vi "ConfChannelMetodo.vi"(7 "Enable Channel (True)":bool=TRUE, 8 "error in (no error)":errorcluster, 10 "ConfigChannel":T1={"Probe Attenuation (10: 10X)"=10, "Vertical Range (10.0 V/div)"=10.0, "Vertical Offset (0.0 divs)"=0.0, "Bandwidth (0: MAX Bandwidth)"=0, "Channel (0: Channel 1)"=0, "Vertical Coupling (1: DC)"=1} {"Vertical Coupling (1: DC)" items=["AC", "DC", "Ground"]; "Channel (0: Channel 1)" items=["Channel 1", "Channel 2", "Channel 3", "Channel 4", "Math", "Reference A", "Reference B", "Reference C", "Reference D"]; "Bandwidth (0: MAX Bandwidth)" items=["MAX Bandwidth", "Unlimited"]; "Probe Attenuation (10: 10X)" items=["1"=1, "10"=10, "20"=20, "50"=50, "100"=100, "500"=500, "1000"=1000]}, 11 "Keysight in":refnum<class "Keysight.lvclass">) -> (0 "error out":errorcluster, 3 "Keysight out":refnum<class "Keysight.lvclass">)   [LabVIEW 2020, in "Keysight.lvclass"]
uses:
  Keysight.lvclass
  Keysight.lvclass/Keysight.ctl
  <instrlib>/Agilent 2000 3000 X-Series/Agilent 2000 3000 X-Series.lvlib
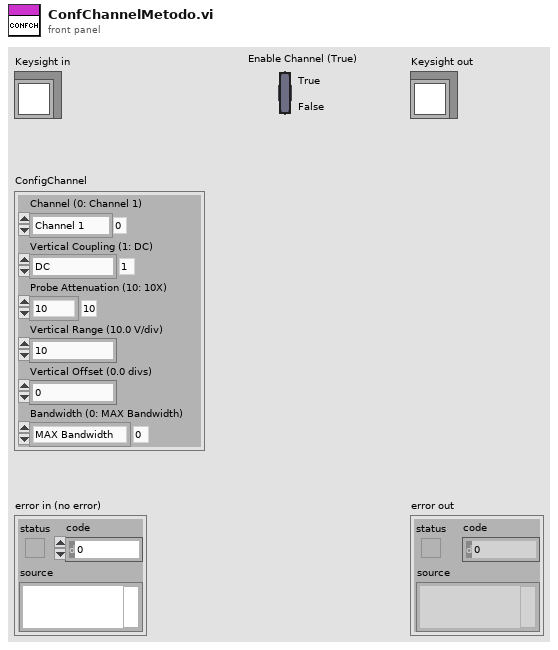
[diagram p1: front panel]
types:
  T1 = cluster{"Probe Attenuation (10: 10X)":i32, "Vertical Range (10.0 V/div)":dbl, "Vertical Offset (0.0 divs)":dbl, "Bandwidth (0: MAX Bandwidth)":i32, "Channel (0: Channel 1)":i32, "Vertical Coupling (1: DC)":i32}
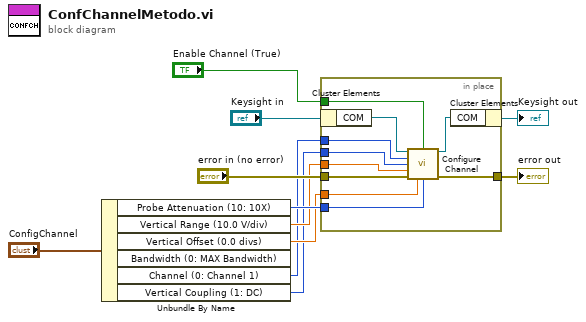
[diagram p0: block diagram]
diagram:
  n1 = Unbundle By Name("ConfigChannel") -> ("Probe Attenuation (10: 10X)"=w5:i32, "Vertical Range (10.0 V/div)"=w4:dbl, "Vertical Offset (0.0 divs)"=w3:dbl, "Channel (0: Channel 1)"=w2:i32, "Vertical Coupling (1: DC)"=w1:i32)  [unwired: 1 out]
  n2 = in-place {
    in-place-border: "Enable Channel (True)" -> [w21]
    in-place-border: [w20] -> w7
    in-place-border: "error in (no error)" -> [w19]
    in-place-border: w5 -> [w18]
    in-place-border: w4 -> [w17]
    in-place-border: w3 -> [w16]
    in-place-border: w2 -> [w15]
    in-place-border: w1 -> [w14]
    n3 = in-place-cluster #1("Keysight in") -> ("COM"=w13:refnum<visa-resource-name>)
    n4 = call <instrlib>:"Configure Channel.vi"("VISA resource name"=w13, "Enable Channel (T: Enable)"=w21, "Channel Name (0: Channel 1)"=w15, "Coupling (1: DC)"=w14, "Vertical Range (40.0 V)"=w17, "error in (no error)"=w19, "Vertical Offset (0.0)"=w16, "Probe Attenuation (1.0)"=w18) -> ("VISA resource name out"=w12:refnum<visa-resource-name>, "error out"=w20:errorcluster)  [unwired: 6 in]
    n5 = in-place-cluster #1("COM"=w12) -> (→"Keysight out":refnum<class "Keysight.lvclass">)
  }
  "error out" <- w7
